vi "Get Result.vi"(6 "Last request":bool, 8 "error in (no error)":errorcluster, 11 "Keithley 622x2182 Driver in":refnum<class "Keithley 622x2182 Driver.lvclass">) -> (0 "error out":errorcluster, 2 "Result":refnum<class "Acquired Result.lvclass">, 3 "Keithley 622x2182 Driver out":refnum<class "Keithley 622x2182 Driver.lvclass">)   [LabVIEW 2021, in "Keithley 622x2182 Driver.lvclass"]
uses:
  Keithley 622x2182 Driver.lvclass
  C:/GitHub/NHMFL_Core/Libraries/Instruments/VISA Instrument/VISA Instrument.lvclass
  Results/Acquired Result/Acquired Result.lvclass
  Results/Combined Result/Combined Result.lvclass
  C:/GitHub/NHMFL_Core/Libraries/Instruments/Results/Acquired Result/Acquired Result.lvclass
  VISA Instrument/VISA Instrument.lvclass/VISA Instrument.ctl
  Keithley 622x2182 Driver.lvclass/Keithley 622x2182 Driver.ctl
  Results/Acquired Result/Acquired Result.lvclass/Acquired Result.ctl
  VISA Instrument/Read VISA resource.vi
  VISA Instrument/Write VISA resource.vi
  Results/Acquired Result/Write Channels.vi
  Results/Acquired Result/Write Group.vi
  <vilib>/express/express shared/transition.llb/Dynamic To Waveform Array.vi
  <vilib>/express/express signal manip/GetorSetDDTAttributes/Set DDT Attributes/SetT0.vi
  <vilib>/express/express shared/transition.llb/Waveform Array To Dynamic.vi
  <vilib>/express/express signal manip/GetorSetDDTAttributes/Set DDT Attributes/Set DDT Properties.xnode
panel:
  out "x/y":dbl
  out "size(s)":i32
  out "Waveform Graph":dbl[](graph)
  out "read buffer":string
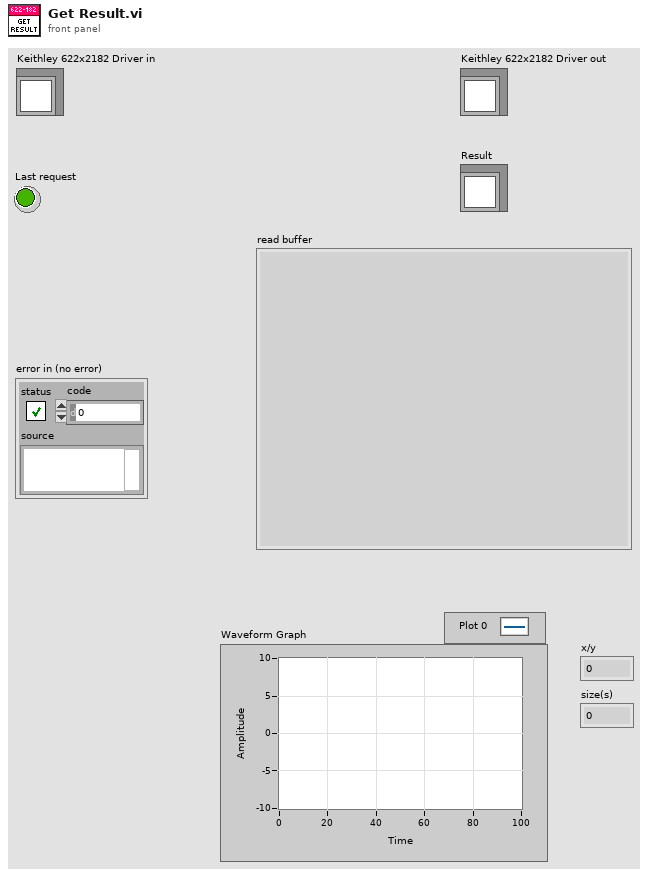
[diagram p1: front panel]
types:
  T1 = typedef "Stepper Config.ctl" = cluster{"Start":dbl, "End":dbl, "Step":dbl, "Delta":dbl, "Scan shape":enum16{"Sawtooth", "Triangular"}, "Append measurements":string[], "Pulse width":dbl, "Pulse interval":dbl, "Scan mode":enum16{"Delta", "Diff. conductance", "Pulse delta sweep"}}
  T2 = enum16{"Delta", "Diff. conductance", "Pulse delta sweep"}
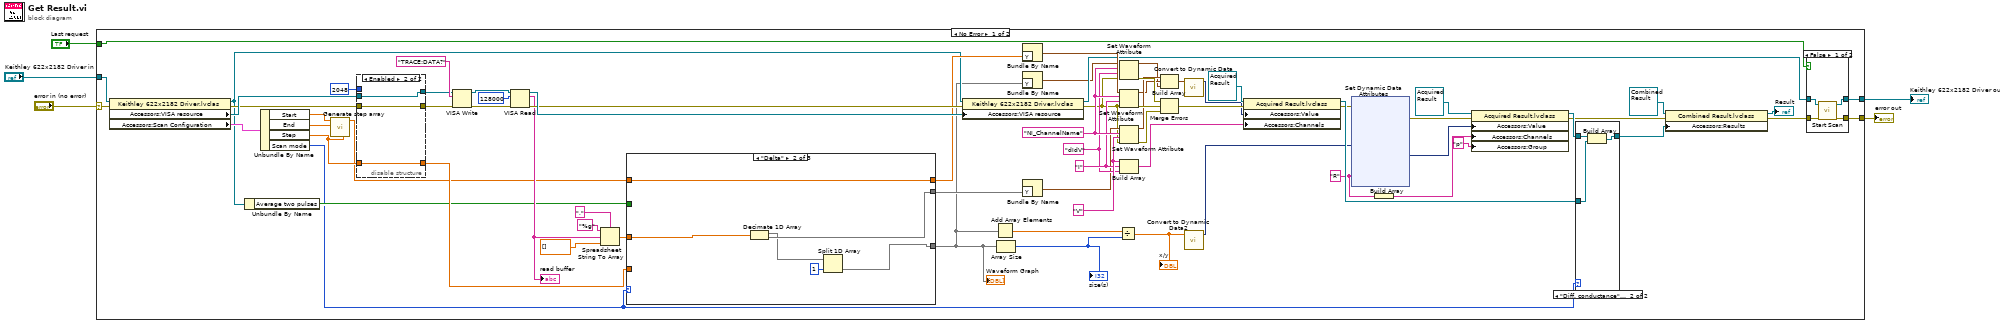
[diagram p0: block diagram]
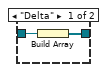
[diagram p2: hidden frame]
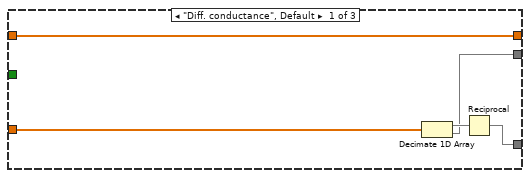
[diagram p4: hidden frame]
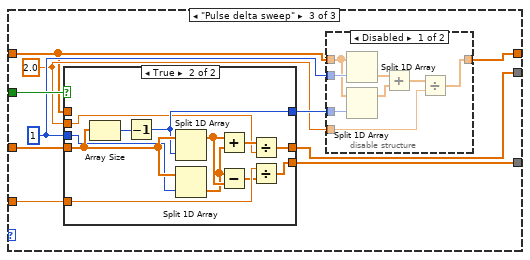
[diagram p5: hidden frame]
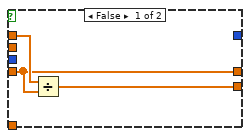
[diagram p6: hidden frame]
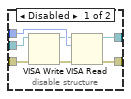
[diagram p8: hidden frame]
diagram:
  n1 = case shown="No Error" "error in (no error)" {
    selector: "error in (no error)" -> [w20 w158]
    tunnel: "Keithley 622x2182 Driver in" -> [w62 w157]
    tunnel: [w40 w157] -> w4
    tunnel: [w22 w158] -> w3
    tunnel: "Last request" -> [w15 _]
    frame No Error {
      w28 = "R" ("String")
      w43 = "I" ("name")
      w44 = "V" ("name")
      w39 = "dIdV" ("name")
      w54 = "NI_ChannelName" ("name")
      n2 = property class="Keithley 622x2182 Driver.lvclas"(reference=w62, error in=w20) -> (reference out=w14:refnum<class "Keithley 622x2182 Driver.lvclass">, error out=w64:errorcluster, "Accessors:VISA resource"=w65:refnum<visa-resource-name>, "Accessors:Scan Configuration"=w59:T1)
      n3 = Unbundle By Name(w14) -> ("Average two pulses"=w13:bool)
      n4 = Unbundle By Name(w59) -> ("Start"=w58:dbl, "End"=w57:dbl, "Step"=w19:dbl, "Scan mode"=w11:T2)
      n5 = call "Generate step array.vi"("Step"=w19, "End"=w57, "Start"=w58) -> ("Steps"=w17:dbl[])  [unwired: 8 in]
      n6 = disable-structure shown="Enabled" {
        disable-tunnel: u32 2048 ("byte count") -> [w153 _]
        disable-tunnel: [w150 w156] -> w66
        disable-tunnel: w65 -> [w149 w155]
        disable-tunnel: w64 -> [w148 w156]
        disable-tunnel: [w147 w155] -> w63
        disable-tunnel: w19 -> [_ w154]
        disable-tunnel: [_ w154] -> w18
        frame Disabled {
          n7 = VISA Write(VISA resource name=w149, error in (no error)=w148) -> (VISA resource name out=w152:refnum<visa-resource-name>, error out=w151:errorcluster)  [unwired: 1 in, 1 out]
          n8 = VISA Read(VISA resource name=w152, byte count=w153, error in (no error)=w151) -> (VISA resource name out=w147:refnum<visa-resource-name>, error out=w150:errorcluster)  [unwired: 2 out]
        }
        frame Enabled {
        }
      }
      n9 = VISA Write(VISA resource name=w63, write buffer="TRACE:DATA?", error in (no error)=w66) -> (VISA resource name out=w74:refnum<visa-resource-name>, error out=w75:errorcluster)  [unwired: 1 out]
      n10 = VISA Read(VISA resource name=w74, byte count=u32 128000, error in (no error)=w75) -> (VISA resource name out=w72:refnum<visa-resource-name>, read buffer=w70:string, error out=w71:errorcluster)  [unwired: 1 out]
      "read buffer" <- w70
      n11 = Spreadsheet String To Array(delimiter (Tab)=",", format string="%g", spreadsheet string=w70, array type (2D Dbl)=dbl[] []) -> (array=w60:dbl[])
      n12 = case shown="\"Delta\"" w11 {
        tunnel: w60 -> [w92 w98 w108]
        tunnel: [w88 w94 w106] -> w6
        tunnel: [w90 w97 w105] -> w21
        tunnel: w17 -> [w89 w96 w99]
        tunnel: w18 -> [_ _ w107]
        tunnel: [w89 w96 w103] -> w16
        tunnel: w13 -> [_ _ w102]
        frame "Diff. conductance", Default {
          n13 = Decimate 1D Array(w92) -> (w91:dbl[], w90:dbl[])
          n14 = Reciprocal(x=w91) -> (1/x=w88:dbl[])
        }
        frame "Delta" {
          n15 = Decimate 1D Array(w98) -> (w95:dbl[], w97:dbl[])
          n16 = Split 1D Array(array=w95, index=1) -> (second subarray=w94:dbl[])  [unwired: 1 out]
        }
        frame "Pulse delta sweep" {
          w100 = 2.0
          w101 = 1 ("index")
          n17 = case shown="True" w102 {
            tunnel: w108 -> [w110 w122]
            tunnel: w107 -> [_ w121]
            tunnel: [w109 w119] -> w106
            tunnel: [w110 w115] -> w105
            tunnel: [_ w114] -> w104
            tunnel: w101 -> [_ w113]
            tunnel: w100 -> [_ w112]
            tunnel: w99 -> [w111 _]
            frame False {
              n18 = Divide(x=w111, y=w110) -> (x/y=w109:dbl[])
            }
            frame True {
              n19 = Array Size(array=w122) -> (size(s)=w123:i32)
              n20 = Decrement(x=w123) -> (x-1=w114:i32)
              n21 = Split 1D Array(array=w122, index=w114) -> (first subarray=w118:dbl[])  [unwired: 1 out]
              n22 = Split 1D Array(array=w122, index=w113) -> (second subarray=w117:dbl[])  [unwired: 1 out]
              n23 = Add(x=w118, y=w117) -> (x+y=w116:dbl[])
              n24 = Subtract(x=w117, y=w118) -> (x-y=w120:dbl[])
              n25 = Divide(x=w116, y=w112) -> (x/y=w115:dbl[])
              n26 = Divide(x=w121, y=w120) -> (x/y=w119:dbl[])
            }
          }
          n27 = disable-structure shown="Disabled" {
            disable-tunnel: w101 -> [w131 _]
            disable-tunnel: w104 -> [w130 _]
            disable-tunnel: w99 -> [w129 w132]
            disable-tunnel: w100 -> [w125 _]
            disable-tunnel: [w124 w132] -> w103
            frame Disabled {
              n28 = Split 1D Array(array=w129, index=w131) -> (second subarray=w128:dbl[])  [unwired: 1 out]
              n29 = Split 1D Array(array=w129, index=w130) -> (first subarray=w127:dbl[])  [unwired: 1 out]
              n30 = Add(x=w128, y=w127) -> (x+y=w126:dbl[])
              n31 = Divide(x=w126, y=w125) -> (x/y=w124:dbl[])
            }
            frame Enabled {
            }
          }
        }
      }
      "Waveform Graph" <- w6
      n32 = property class="Keithley 622x2182 Driver.lvclas"(reference=w14, error in=w71, "Accessors:VISA resource"=w72) -> (reference out=w41:refnum<class "Keithley 622x2182 Driver.lvclass">, error out=w23:errorcluster)
      n33 = Add Array Elements(numeric array=w6) -> (sum=w36:dbl)
      n34 = Array Size(array=w6) -> (size(s)=w35:i32)
      "size(s)" <- w35
      n35 = Bundle By Name("Y"=w16) -> (w55:waveform(dbl))  [unwired: 1 in]
      n36 = Bundle By Name("Y"=w6) -> (w38:waveform(dbl))  [unwired: 1 in]
      n37 = Bundle By Name("Y"=w21) -> (w37:waveform(dbl))  [unwired: 1 in]
      n38 = Divide(x=w36, y=w35) -> (x/y=w12:dbl)
      "x/y" <- w12
      n39 = Set Waveform Attribute(4:w23, 5:w39, 6:w54, 7:w38) -> (0:w53:errorcluster, 3:w47:waveform(dbl))  [unwired: 1 out]
      n40 = Set Waveform Attribute(4:w23, 5:w43, 6:w54, 7:w55) -> (0:w52:errorcluster, 3:w48:waveform(dbl))  [unwired: 1 out]
      n41 = Set Waveform Attribute(4:w23, 5:w44, 6:w54, 7:w37) -> (0:w51:errorcluster, 3:w49:waveform(dbl))  [unwired: 1 out]
      n42 = Build Array(w44, w43, w39) -> (w42:string[])
      n43 = Build Array(w49, w48, w47) -> (w46:waveform(dbl)[])
      n44 = Merge Errors(w53, w52, w51) -> (w50:errorcluster)
      n45 = call "Convert to Dynamic Data"("Array of Waveforms"=w46) -> ("Dynamic Data Type"=w45:dynamicdata)  [unwired: 3 in]
      n46 = call "Convert to Dynamic Data2"("Double"=w12) -> ("Dynamic Data Type"=w29:dynamicdata)  [unwired: 3 in]
      n47 = property class="Acquired Result.lvclass"(reference=refnum<class "Acquired Result.lvclass"> refnum ("Result"), error in=w50, "Accessors:Value"=w45, "Accessors:Channels"=w42) -> (reference out=w32:refnum<class "Acquired Result.lvclass">, error out=w25:errorcluster)
      n48 = xnode "Set Dynamic Data Attributes"("Signals In"=w29, "Signal Name"=w28, "error in"=w25) -> ("Signals Out"=w26:dynamicdata, "error out"=w24:errorcluster)  [unwired: 1 in]
      n49 = Build Array(w28) -> (w27:string[])
      n50 = property class="Acquired Result.lvclass"(reference=refnum<class "Acquired Result.lvclass"> refnum ("Result"), error in=w24, "Accessors:Value"=w26, "Accessors:Channels"=w27, "Accessors:Group"="p" ("Group")) -> (reference out=w33:refnum<class "Acquired Result.lvclass">, error out=w31:errorcluster)
      n51 = case shown="\"Diff. conductance\", Default" w11 {
        tunnel: w33 -> [w78 w81]
        tunnel: w32 -> [_ w80]
        tunnel: [w77 w79] -> w10
        frame "Delta" {
          n52 = Build Array(w78) -> (w77:refnum<class "Acquired Result.lvclass">[])
        }
        frame "Diff. conductance", Default {
          n53 = Build Array(w81, w80) -> (w79:refnum<class "Acquired Result.lvclass">[])
        }
      }
      n54 = property class="Combined Result.lvclass"(reference=refnum<class "Combined Result.lvclass"> refnum ("Combined Result.lvclass"), error in=w31, "Accessors:Results"=w10) -> (reference out=→"Result":refnum<class "Combined Result.lvclass">, error out=w8:errorcluster)
      n55 = case shown="False" w15 {
        tunnel: w41 -> [w85 w87]
        tunnel: [w84 w87] -> w40
        tunnel: w8 -> [w83 w86]
        tunnel: [w82 w86] -> w22
        frame False {
          n56 = call-dynamic "Start Scan.vi"("error in (no error)"=w83, "Keithley 622x2182 Driver in"=w85) -> ("error out"=w82:errorcluster, "Keithley 622x2182 Driver out"=w84:refnum<class "Keithley 622x2182 Driver.lvclass">)  [unwired: 8 in]
        }
        frame True {
        }
      }
    }
    frame Error {
    }
  }
  "error out" <- w3
  "Keithley 622x2182 Driver out" <- w4
